vi "Scale Instructions.vi"(1 "Scale":i16, 2 "Instructions":i32[][](array[numeric])) -> (0 "Scaled Instructions":i32[][](array[numeric]))   [LabVIEW 2015]
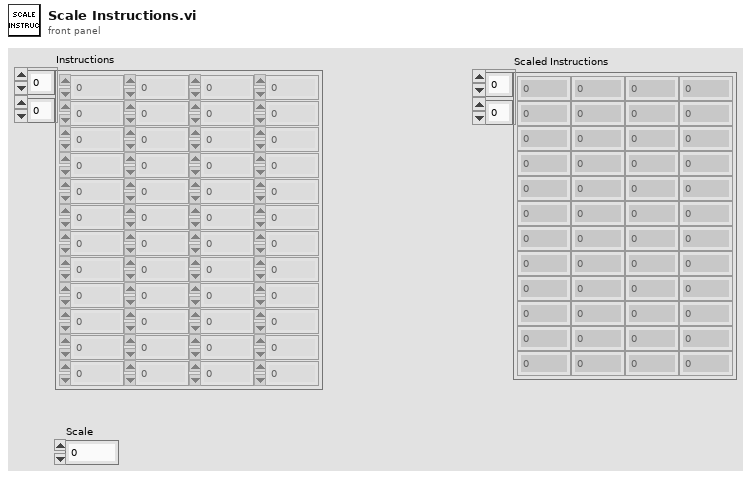
[diagram p1: front panel]
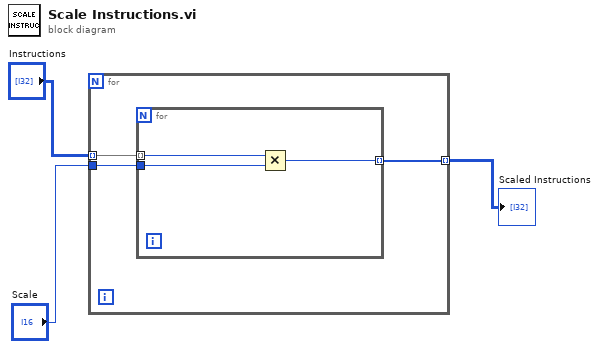
[diagram p0: block diagram]
diagram:
  n1 = for {
    tunnel: "Scale" -> [w6]
    tunnel: "Instructions" -> [w5] mode=indexing
    tunnel: [w4] -> w1 mode=indexing
    n2 = for {
      tunnel: w6 -> [w9]
      tunnel: w5 -> [w8] mode=indexing
      tunnel: [w7] -> w4 mode=indexing
      n3 = Multiply(x=w8, y=w9) -> (x*y=w7:i32)
    }
  }
  "Scaled Instructions" <- w1
